vi "Test App Get Nested Process by Qualified Name.vi"(8 "error in (no error)":errorcluster, 11 "Application Test in":refnum<class "Application Test.lvclass">) -> (0 "error out":errorcluster, 3 "Application Test out":refnum<class "Application Test.lvclass">)   [LabVIEW 2020, in "Application Test.lvclass"]
uses:
  Application Test.lvclass
  C:/Program Files (x86)/National Instruments/LabVIEW 2020/vi.lib/Asteme/LUnit/Test Case.lvclass
  Framework/Process/Process.lvclass
  Framework/Process/Process.lvclass/Process.ctl
  Framework/Application/Application.lvclass/Application.ctl
  <vilib>/Asteme/LUnit/Test Case.lvclass/Test Case.ctl
  <vilib>/Asteme/LUnit/LUnit Assertion Result.lvclass/LUnit Assertion Result.ctl
  Framework/Application/Private/Add Process to Map.vi
  Framework/Application/Private/Start Idle Processes if Running.vi
  Framework/Process/Protected/Messaging/Enqueue Message.vi
  Framework/Process/Public/Lifecycle/Get Lifecycle State.vi
  Framework/Process/Protected/SubVIs/Set Context.vi
  Framework/Process/Protected/Messaging/Request Message.vi
  <vilib>/Asteme/LUnit/Palette/Pass.vi
  <vilib>/Asteme/LUnit/Palette/Fail.vi
  <vilib>/Asteme/LUnit/Set Assertion Type.vi
  Framework/Process/Private/SubVIs/Wait for finish.vi
  Framework/Process/Private/SubVIs/Set Lifecycle State.vi
  <vilib>/Utility/error.llb/Clear Errors.vi
  Framework/Process/Public/Lifecycle/Leave Process Loop.vi
  Framework/Process/Private/SubVIs/Enqueue Request Message.vi
  <vilib>/Asteme/LUnit/Add test result.vi
  <vilib>/Asteme/LUnit/LUnit Write Passed.vi
  <vilib>/Asteme/LUnit/LUnit Get Test Case.vi
  <vilib>/Asteme/LUnit/Assertion Result/LUnit Get Test Name.vi
  <vilib>/Asteme/LUnit/LUnit Write Message.vi
  <vilib>/Asteme/LUnit/LUnit Write Description.vi
  <vilib>/Asteme/LUnit/LUnit Write Assertion Type.vi
  <vilib>/Asteme/LUnit/Read Test Case Name.vi
  Framework/Application/Application.lvclass
  C:/Users/anton/Documents/GitHub/Triarc-Framework/source/Framework/Process/Process.lvclass
  <vilib>/Utility/error.llb/Error Cluster From Error Code.vi
  Framework/Application/Private/Update Context for Owned Processes.vi
  Framework/Process/Private/SubVIs/Wait for Response Message.vi
  <vilib>/Asteme/LUnit/LUnit Assertion Result.lvclass
  <vilib>/Asteme/LUnit/Test Case.lvclass
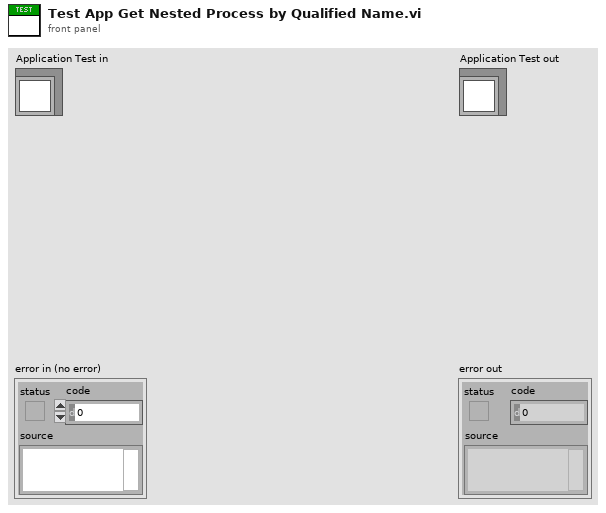
[diagram p1: front panel]
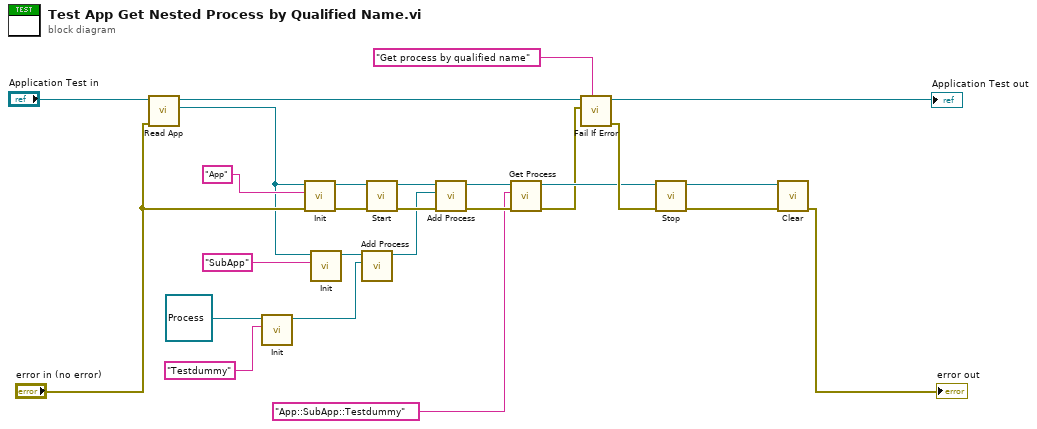
[diagram p0: block diagram]
diagram:
  n1 = call "Read App.vi"("error in (no error)"="error in (no error)", "Application Test In"="Application Test in") -> ("App out"=w5:refnum<class "Application.lvclass">, "Application Test Out"=w26:refnum<class "Application Test.lvclass">)  [unwired: 7 in, 1 out]
  n2 = call-dynamic "Init.vi"("Name"="Testdummy", "Process In"=refnum<class "Process.lvclass"> refnum ("Process.lvclass")) -> ("Process Out"=w1:refnum<class "Process.lvclass">)  [unwired: 8 in, 1 out]
  n3 = call-dynamic "Init.vi"("error in (no error)"="error in (no error)", "Name"="App", "Process In"=w5) -> ("error out"=w24:errorcluster, "Process Out"=w25:refnum<class "Application.lvclass">)  [unwired: 7 in]
  n4 = call-dynamic "Init.vi"("Name"="SubApp", "Process In"=w5) -> ("Process Out"=w3:refnum<class "Application.lvclass">)  [unwired: 8 in, 1 out]
  n5 = call "Add Process.vi"("Process"=w1, "Rig In"=w3) -> ("Rig Out"=w2:refnum<class "Application.lvclass">)  [unwired: 8 in, 1 out]
  n6 = call "Start.vi"("error in (no error)"=w24, "Process In"=w25) -> ("error out"=w21:errorcluster, "Process Out"=w9:refnum<class "Application.lvclass">)  [unwired: 8 in]
  n7 = call "Add Process.vi"("error in (no error)"=w21, "Process"=w2, "Rig In"=w9) -> ("error out"=w22:errorcluster, "Rig Out"=w10:refnum<class "Application.lvclass">)  [unwired: 7 in]
  n8 = call "Get Process.vi"("error in (no error)"=w22, "Process Name"="App::SubApp::Testdummy" ("Name"), "Rig In"=w10) -> ("error out"=w6:errorcluster, "Rig Out"=w8:refnum<class "Application.lvclass">)  [unwired: 6 in, 1 out]
  n9 = call <vilib>:"Fail If Error.vi"("Description"="Get process by qualified name", "Assert error"=w6, "Test Case In"=w26) -> ("error out"=w18:errorcluster, "Test Case Out"=→"Application Test out":refnum<class "Application Test.lvclass">)  [unwired: 7 in]
  n10 = call "Stop.vi"("error in (no error)"=w18, "Process In"=w8) -> ("error out"=w15:errorcluster, "Process Out"=w23:refnum<class "Application.lvclass">)  [unwired: 7 in, 1 out]
  n11 = call-dynamic "Clear.vi"("error in (no error)"=w15, "Application In"=w23) -> ("error out"=→"error out":errorcluster)  [unwired: 9 in]
